vi "Begin.vi"(8 "error in":errorcluster) -> (0 "error out":errorcluster)   [LabVIEW 2016]
doc: "Called before other user functions, this VI is expected to open initial I/O refnums, load in file data, and do all program initialization. Notice that the <B>error out</B> terminal is simply used for data flow. Wiring it to other structures or subVIs ensures that this VI runs first."
uses:
  <vilib>/Rock Robotics/WPI/DriverStation/WPI_DriverStationRobotMode2.ctl
  <vilib>/Rock Robotics/WPI/ThirdParty/CanMotor/TalonSRX/WPI_CANTalonSRX_APIControlMode.ctl
  <vilib>/Rock Robotics/SystemInterfaces/DIO/FPGA_DIOPWMChannel.ctl
  <vilib>/Rock Robotics/SystemInterfaces/AI/FPGA_AIChannel.ctl
  <vilib>/Rock Robotics/WPI/AnalogOutput/WPI_AnalogOutputChannel.ctl
  Robot Global Data.vi
  <vilib>/Rock Robotics/WPI/MotorControl/WPI_MotorControlOpen VictorSP.vi
  <vilib>/Rock Robotics/WPI/MotorControl/WPI_MotorControlOpen Talon.vi
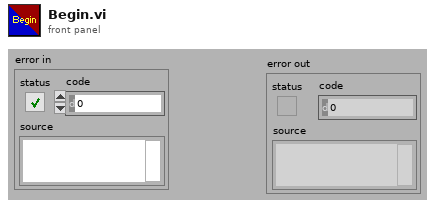
[diagram p1: front panel]
types:
  T1 = typedef "WPI_AnalogOutputChannel.ctl" = enum8{"AO MXP 0", "AO MXP 1", "Invalid"}
  T2 = typedef "FPGA_AIChannel.ctl" = enum8{"AI 0", "AI 1", "AI 2", "AI 3", "AI MXP 0", "AI MXP 1", "AI MXP 2", "AI MXP 3", "Invalid"}
  T3 = typedef "FPGA_DIOPWMChannel.ctl" = enum8{"PWM 0", "PWM 1", "PWM 2", "PWM 3", "PWM 4", "PWM 5", "PWM 6", "PWM 7", "PWM 8", "PWM 9", "PWM MXP 0", "PWM MXP 1", "PWM MXP 2", "PWM MXP 3", "PWM MXP 4", "PWM MXP 5", "PWM MXP 6", "PWM MXP 7", "PWM MXP 8", "PWM MXP 9", "Invalid"}
  T4 = typedef "WPI_CANTalonSRX_APIControlMode.ctl" = enum8{"Percent VBus", "Speed", "Position", "Slave", "Unchanged / Invalid", "Voltage Compensation", "Current", "Motion Profile", "Motion Magic"}
  T5 = typedef "WPI_DriverStationRobotMode2.ctl" = enum16{"Autonomous Disabled", "Autonomous Enabled", "Teleop Disabled", "Teleop Enabled", "Disconnected", "Finish", "Test Disabled", "Test Enabled", "Emergency Stopped"}
  T6 = typedef "WPI_AOChannelDevRef.ctl" = cluster{"DevStatus":errorcluster, "AO Channel":T1}
  T7 = typedef "WPI_MotorControlDeviceRef.ctl" = cluster{"DeviceStatus":errorcluster, "Type":T8, "PWM":cluster{"PWM Channel":T3, "DeadBand":T9}, "CAN":cluster{"Device Number":u8, "SetOutput VI Ref":variant, "GetOutput VI Ref":variant, "Enable VI Ref":variant, "Disable VI Ref":variant, "Data":variant}, "Invert":bool}
  T8 = typedef "WPI_MotorControlType.ctl" = enum16{"PWM", "CAN"}
  T9 = typedef "WPI_PWMDeadband.ctl" = cluster{"Name":string, "maxPositivePwm":i32, "minPositivePwm":i32, "centerPwm":i32, "maxNegativePwm":i32, "minNegativePwm":i32, "angularRange":u16}
  T10 = typedef "WPI_PotentiometerDevRef.ctl" = cluster{"DevStatus":errorcluster, "Analog Channel":T2, "Invert Output":bool}
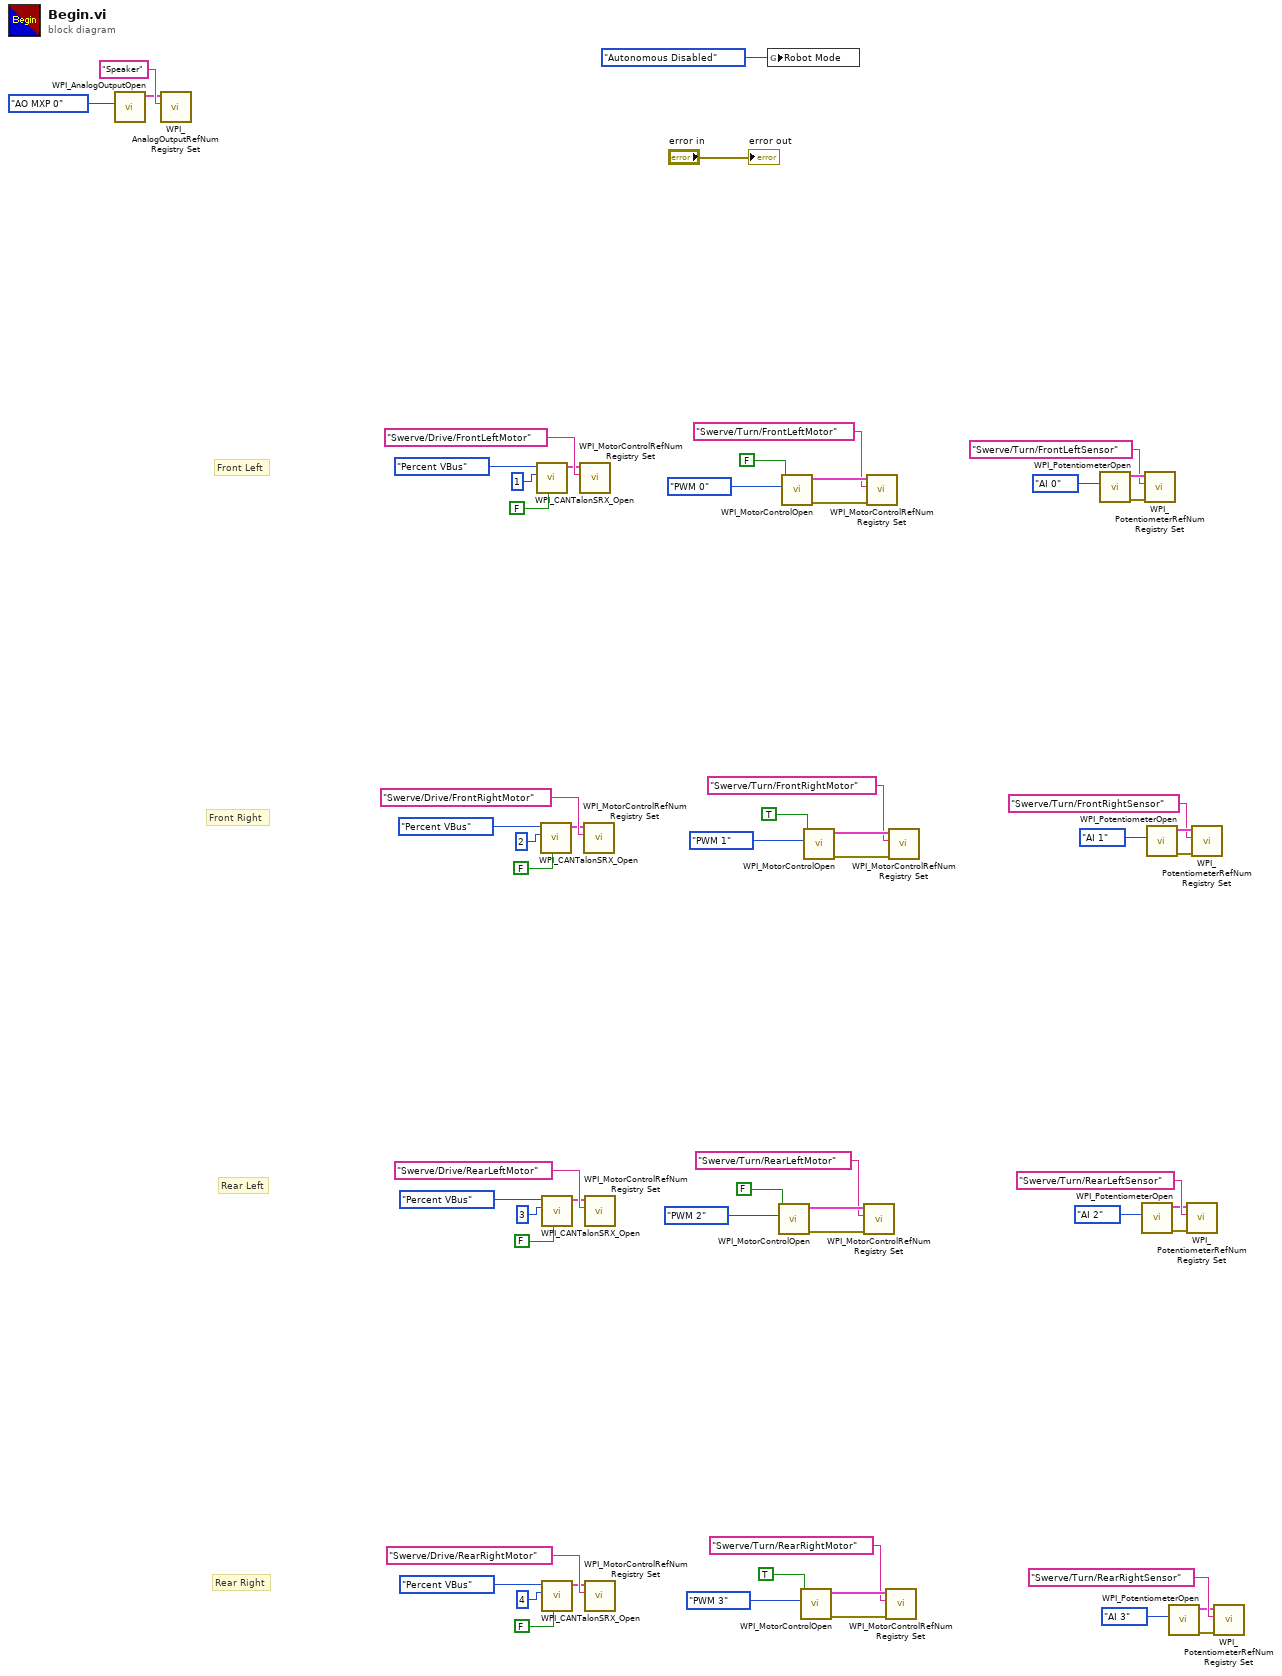
[diagram p0: block diagram]
diagram:
  # "Rear Right"
  # "Rear Left"
  # "Front Right"
  # "Front Left"
  n1 = call <vilib>:"WPI_AnalogOutputOpen.vi"("AO Channel"=WPI_AnalogOutputChannel."AO MXP 0") -> ("AODeviceRef"=w1:T6)  [unwired: 9 in, 1 out]
  n2 = call <vilib>:"WPI_AnalogOutputRefNum Registry Set.vi"("refnum name"="Speaker", "AODeviceRef"=w1) -> ()  [unwired: 8 in, 2 out]
  n3 = call <vilib>:"WPI_CANTalonSRX_Open.vi"("Invert"=FALSE, "Device Number"=u8 1, "Control Mode"=WPI_CANTalonSRX_APIControlMode."Percent VBus") -> ("CAN Talon SRX Ref"=w55:T7)  [unwired: 7 in, 1 out]
  n4 = call <vilib>:"WPI_CANTalonSRX_Open.vi"("Invert"=FALSE, "Device Number"=u8 2, "Control Mode"=WPI_CANTalonSRX_APIControlMode."Percent VBus") -> ("CAN Talon SRX Ref"=w50:T7)  [unwired: 7 in, 1 out]
  n5 = call <vilib>:"WPI_CANTalonSRX_Open.vi"("Invert"=FALSE, "Device Number"=u8 3, "Control Mode"=WPI_CANTalonSRX_APIControlMode."Percent VBus") -> ("CAN Talon SRX Ref"=w45:T7)  [unwired: 7 in, 1 out]
  n6 = call <vilib>:"WPI_CANTalonSRX_Open.vi"("Invert"=FALSE, "Device Number"=u8 4, "Control Mode"=WPI_CANTalonSRX_APIControlMode."Percent VBus") -> ("CAN Talon SRX Ref"=w40:T7)  [unwired: 7 in, 1 out]
  n7 = call <vilib>:"WPI_MotorControlRefNum Registry Set.vi"("refnum name"="Swerve/Drive/FrontLeftMotor", "MotorControlDevRef"=w55) -> ()  [unwired: 8 in, 2 out]
  n8 = call <vilib>:"WPI_MotorControlRefNum Registry Set.vi"("refnum name"="Swerve/Drive/FrontRightMotor", "MotorControlDevRef"=w50) -> ()  [unwired: 8 in, 2 out]
  n9 = call <vilib>:"WPI_MotorControlRefNum Registry Set.vi"("refnum name"="Swerve/Drive/RearLeftMotor", "MotorControlDevRef"=w45) -> ()  [unwired: 8 in, 2 out]
  n10 = call <vilib>:"WPI_MotorControlRefNum Registry Set.vi"("refnum name"="Swerve/Drive/RearRightMotor", "MotorControlDevRef"=w40) -> ()  [unwired: 8 in, 2 out]
  n11 = global write "Robot Global Data.vi" "Robot Mode"(WPI_DriverStationRobotMode2."Autonomous Disabled" ("Robot Mode")) -> ()
  n12 = call-poly <vilib>:"WPI_MotorControlOpen.vi"("Eliminate Deadband"=FALSE ("Left Motor Inverted"), "PWM Channel"=FPGA_DIOPWMChannel."PWM 2" ("Left Motor")) -> ("error out"=w27:errorcluster, "MotorControlDeviceRef"=w30:T7)  [unwired: 8 in]
  n13 = call-poly <vilib>:"WPI_MotorControlOpen.vi"("Eliminate Deadband"=FALSE ("Left Motor Inverted"), "PWM Channel"=FPGA_DIOPWMChannel."PWM 0" ("Left Motor")) -> ("error out"=w9:errorcluster, "MotorControlDeviceRef"=w12:T7)  [unwired: 8 in]
  n14 = call-poly <vilib>:"WPI_MotorControlOpen.vi"("Eliminate Deadband"=TRUE ("Left Motor Inverted"), "PWM Channel"=FPGA_DIOPWMChannel."PWM 3" ("Left Motor")) -> ("error out"=w37:errorcluster, "MotorControlDeviceRef"=w39:T7)  [unwired: 8 in]
  n15 = call-poly <vilib>:"WPI_MotorControlOpen.vi"("Eliminate Deadband"=TRUE ("Left Motor Inverted"), "PWM Channel"=FPGA_DIOPWMChannel."PWM 1" ("Left Motor")) -> ("error out"=w19:errorcluster, "MotorControlDeviceRef"=w21:T7)  [unwired: 8 in]
  n16 = call <vilib>:"WPI_MotorControlRefNum Registry Set.vi"("error in (no error)"=w27, "refnum name"="Swerve/Turn/RearLeftMotor", "MotorControlDevRef"=w30) -> ()  [unwired: 7 in, 2 out]
  n17 = call <vilib>:"WPI_MotorControlRefNum Registry Set.vi"("error in (no error)"=w9, "refnum name"="Swerve/Turn/FrontLeftMotor", "MotorControlDevRef"=w12) -> ()  [unwired: 7 in, 2 out]
  n18 = call <vilib>:"WPI_MotorControlRefNum Registry Set.vi"("error in (no error)"=w37, "refnum name"="Swerve/Turn/RearRightMotor", "MotorControlDevRef"=w39) -> ()  [unwired: 7 in, 2 out]
  n19 = call <vilib>:"WPI_MotorControlRefNum Registry Set.vi"("error in (no error)"=w19, "refnum name"="Swerve/Turn/FrontRightMotor", "MotorControlDevRef"=w21) -> ()  [unwired: 7 in, 2 out]
  n20 = call <vilib>:"WPI_PotentiometerOpen.vi"("Analog Channel"=FPGA_AIChannel."AI 0") -> ("error out"=w6:errorcluster, "PotDevRef"=w7:T10)  [unwired: 9 in]
  n21 = call <vilib>:"WPI_PotentiometerOpen.vi"("Analog Channel"=FPGA_AIChannel."AI 2") -> ("error out"=w23:errorcluster, "PotDevRef"=w22:T10)  [unwired: 9 in]
  n22 = call <vilib>:"WPI_PotentiometerRefNum Registry Set.vi"("error in (no error)"=w6, "refnum name"="Swerve/Turn/FrontLeftSensor", "PotDevRef"=w7) -> ()  [unwired: 7 in, 2 out]
  n23 = call <vilib>:"WPI_PotentiometerOpen.vi"("Analog Channel"=FPGA_AIChannel."AI 1") -> ("error out"=w15:errorcluster, "PotDevRef"=w16:T10)  [unwired: 9 in]
  n24 = call <vilib>:"WPI_PotentiometerOpen.vi"("Analog Channel"=FPGA_AIChannel."AI 3") -> ("error out"=w32:errorcluster, "PotDevRef"=w31:T10)  [unwired: 9 in]
  n25 = call <vilib>:"WPI_PotentiometerRefNum Registry Set.vi"("error in (no error)"=w23, "refnum name"="Swerve/Turn/RearLeftSensor", "PotDevRef"=w22) -> ()  [unwired: 7 in, 2 out]
  n26 = call <vilib>:"WPI_PotentiometerRefNum Registry Set.vi"("error in (no error)"=w15, "refnum name"="Swerve/Turn/FrontRightSensor", "PotDevRef"=w16) -> ()  [unwired: 7 in, 2 out]
  n27 = call <vilib>:"WPI_PotentiometerRefNum Registry Set.vi"("error in (no error)"=w32, "refnum name"="Swerve/Turn/RearRightSensor", "PotDevRef"=w31) -> ()  [unwired: 7 in, 2 out]
  "error out" <- "error in"
